vi "Test.vi"   [LabVIEW 2018]
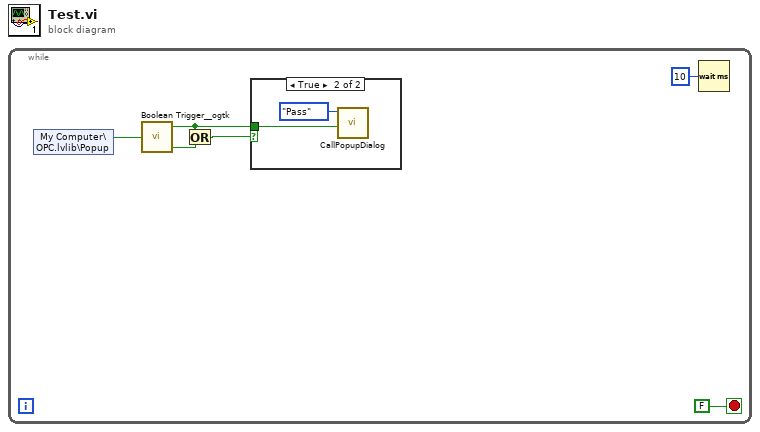
[diagram p0: block diagram]
diagram:
  n1 = while {
    stop <- FALSE stop-if-true
    n2 = shared-variable "My Computer\\OPC.lvlib\\Popup"() -> (w4:bool)  [unwired: 1 in, 1 out]
    n3 = call <userlib>:"Boolean Trigger__ogtk.vi"("Boolean Input"=w4) -> ("Rising Edge"=w1:bool, "Falling Edge"=w3:bool)  [unwired: 1 in]
    n4 = Or(x=w1, y=w3) -> (x .or. y?=w2:bool)
    n5 = case shown="True" w2 {
      tunnel: w1 -> [_ w7]
      frame False {
      }
      frame True {
        n6 = call "CallPopupDialog.vi"("Open/Close"=w7, "Enum"=enum16{"Pass", "Fail", "Error"}."Pass") -> ()  [unwired: 10 in]
      }
    }
    n7 = Wait (ms)(milliseconds to wait=u32 10) -> ()  [unwired: 1 out]
  }
